vi "Read Serial Poll Status.vi"(8 "error in":errorcluster, 11 "SR 3XX HVPS in":refnum<class "SR 3XX HVPS.lvclass">) -> (0 "error out":errorcluster, 2 "SerialPollStat":T1, 3 "SR 3XX HVPS out":refnum<class "SR 3XX HVPS.lvclass">)   [LabVIEW 2014, in "SR 3XX HVPS.lvclass"]
doc: "The *STB? common query reads the value of the serial poll byte. Reading this register has no effect on its value. It is just the summary of the other status registers. The output byte is defined in the cluster <B>SerialPollStat</B>.s"
uses:
  SR 3XX HVPS.lvclass
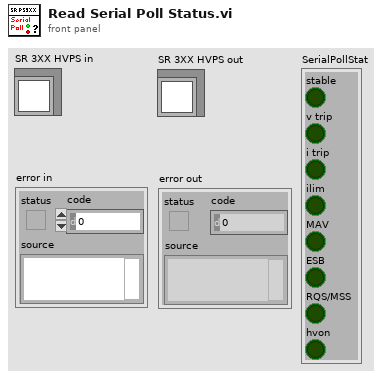
[diagram p1: front panel]
types:
  T1 = cluster{"stable":bool, "v trip":bool, "i trip":bool, "ilim":bool, "MAV":bool, "ESB":bool, "RQS/MSS":bool, "hvon":bool}
  T2 = cluster{"Boolean array[0]":bool, "Boolean array[1]":bool, "Boolean array[2]":bool, "Boolean array[3]":bool, "Boolean array[4]":bool, "Boolean array[5]":bool, "Boolean array[6]":bool, "Boolean array[7]":bool}
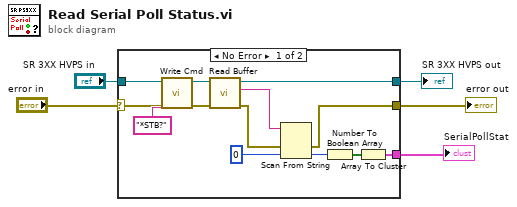
[diagram p0: block diagram]
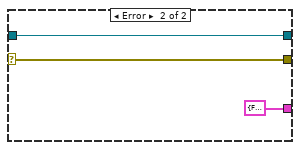
[diagram p2: hidden frame]
diagram:
  n1 = case shown="No Error" "error in" {
    selector: "error in" -> [w16 w21]
    tunnel: [w8 w21] -> w4
    tunnel: [w13 w20] -> w2
    tunnel: "SR 3XX HVPS in" -> [w18 w20]
    tunnel: [w6 T2 {"Boolean array[0]"=FALSE, "Boolean array[1]"=FALSE, "Boolean array[2]"=FALSE, "Boolean array[3]"=FALSE, "Boolean array[4]"=FALSE, "Boolean array[5]"=FALSE, "Boolean array[6]"=FALSE, "Boolean array[7]"=FALSE} ("Boolean array")] -> w1
    frame No Error {
      n2 = call "Write Cmd.vi"("error in"=w16, "Cmd"="*STB?", "SR 3XX HVPS in"=w18) -> ("error out"=w14:errorcluster, "SR 3XX HVPS out"=w15:refnum<class "SR 3XX HVPS.lvclass">)  [unwired: 7 in]
      n3 = call "Read Buffer.vi"("error in"=w14, "SR 3XX HVPS in"=w15) -> ("error out"=w9:errorcluster, "ReadData"=w12:string, "SR 3XX HVPS out"=w13:refnum<class "SR 3XX HVPS.lvclass">)  [unwired: 7 in]
      n4 = Scan From String(input string=w12, error in=w9, default 1=u8 0 ("default value 1")) -> (error out=w8:errorcluster, output 1=w10:u8)  [unwired: 2 in, 2 out]
      n5 = Number To Boolean Array(number=w10) -> (Boolean array=w7:bool[])
      n6 = Array To Cluster(array=w7) -> (cluster=w6:T2)
    }
    frame Error {
    }
  }
  "error out" <- w4
  "SR 3XX HVPS out" <- w2
  "SerialPollStat" <- w1
